vi "RS232SerialTest.vi"() -> ()   [LabVIEW 2016]
uses:
  <vilib>/FPGAPlugInAG/cRIO-9038/niLvFpga_Open_cRIO-9038.vi
  <vilib>/rvi/interface/common/dynamic/niFpgaDynamicAddResources.vi
  <vilib>/FPGAPlugInAG/Dynamic/niLvFpga_Abort_Dynamic.vi
  <vilib>/FPGAPlugInAG/Dynamic/niLvFpga_Reset_Dynamic.vi
  <vilib>/FPGAPlugInAG/Dynamic/niLvFpga_Run_Dynamic.vi
  <vilib>/Utility/error.llb/Error Cluster From Error Code.vi
  <vilib>/rvi/errors/niLvFpgaAdjustHostInterfaceError.vi
  <vilib>/FPGAPlugInAG/Dynamic/niLvFpga_Close_Dynamic.vi
  <vilib>/rvi/interface/nirviOpenFPGA/nirviOpenFPGA.xnode
  FPGA Bitfiles/Modbus_FPGATarget_RS232SerialPortT_8rmEXQNE11k.lvbitx
  RS232SerialPortTest.vi
  <vilib>/rvi/interface/nirviMethod/nirviMethod.xnode
  <vilib>/rvi/interface/nirviCloseFPGA/nirviCloseFPGA.xnode
  <vilib>/rvi/errors/niLvFpgaMergeErrorWithErrorCode.vi
  <vilib>/FPGAPlugInAG/Dynamic/niLvFpga_ReadFifo_Dynamic.vi
  <vilib>/FPGAPlugInAG/Dynamic/niLvFpga_WriteFifo_Dynamic.vi
panel:
  out "Receive":u64[](array[numeric]) format="%02x"
  in  "Send":u64[](array[numeric])=[127, 3, 0, 0, 0, 2, 206, 21] format="%02x"
  in  "Send":bool
  in  "Stop":bool
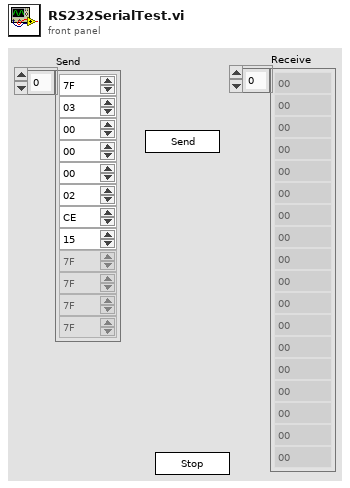
[diagram p1: front panel]
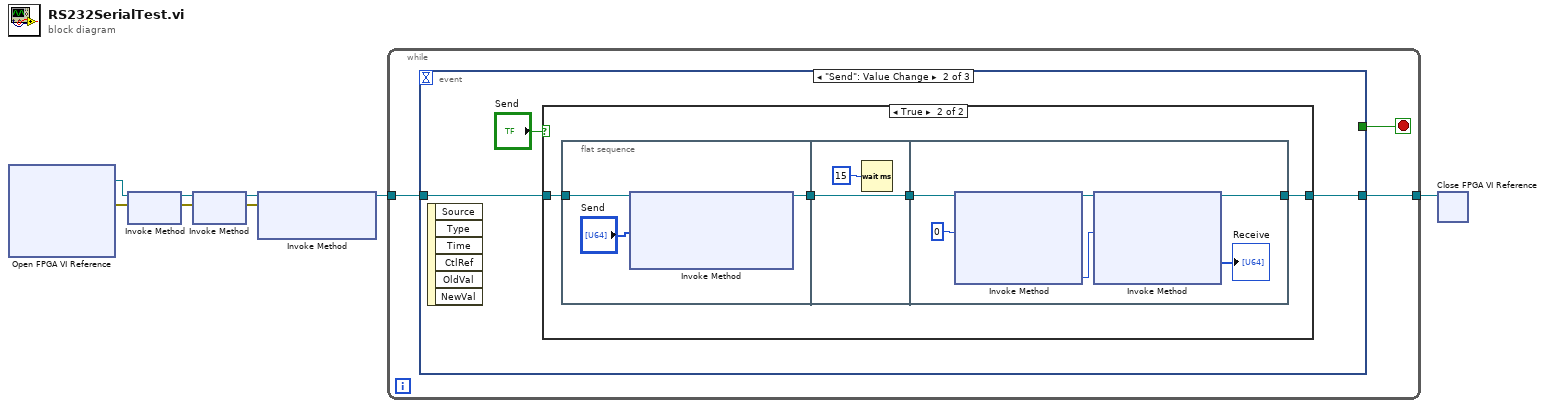
[diagram p0: block diagram]
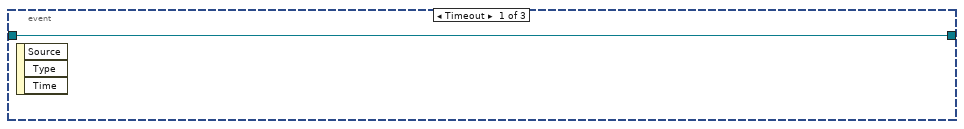
[diagram p2: hidden frame]
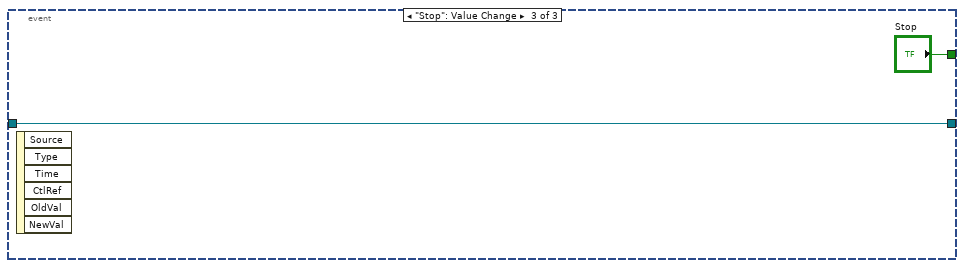
[diagram p4: hidden frame]
diagram:
  n1 = xnode "Open FPGA VI Reference"() -> ("FPGA VI Reference Out"=w8:refnum<k20>, "error out"=w5:errorcluster)  [unwired: 2 in]
  n2 = xnode "Invoke Method"("FPGA VI Reference In"=w8, "error in"=w5) -> ("FPGA VI Reference Out"=w7:refnum<k20>, "error out"=w4:errorcluster)
  n3 = xnode "Invoke Method"("FPGA VI Reference In"=w7, "error in"=w4) -> ("FPGA VI Reference Out"=w6:refnum<k20>, "error out"=w3:errorcluster)
  n4 = xnode "Invoke Method"("FPGA VI Reference In"=w6, "error in"=w3) -> ("FPGA VI Reference Out"=w2:refnum<k20>)  [unwired: 1 in, 1 out]
  n5 = while {
    tunnel: w2 -> [w11]
    tunnel: [w9] -> w1
    stop <- w10 stop-if-true
    n6 = event shown="[1] \"Send\": Value Change" {
      selector: _ -> [_ _ _]
      dyn-events: _ -> [_ _ _]
      timeout: _ -> [_ _ _]
      tunnel: w11 -> [w12 w14 w32]
      tunnel: [_ _ "Stop"] -> w10
      tunnel: [w12 w13 w32] -> w9
      event Timeout {
        n7 = event-data() -> ()  [unwired: 1 in, 3 out]
      }
      event "Send": Value Change {
        n8 = event-data() -> ()  [unwired: 1 in, 6 out]
        n9 = case shown="True" "Send" {
          tunnel: w14 -> [w16 w20]
          tunnel: [w16 w17] -> w13
          frame False {
          }
          frame True {
            n10 = flat-sequence {
              tunnel: w20 -> [w22]
              tunnel: [w21] -> w18
              tunnel: [w24] -> w19
              tunnel: w18 -> [w24]
              tunnel: w19 -> [w31]
              tunnel: [w26] -> w17
              frame #0 {
                n11 = xnode "Invoke Method"("FPGA VI Reference In"=w22, "Data"="Send") -> ("FPGA VI Reference Out"=w21:refnum<k20>)  [unwired: 2 in, 2 out]
              }
              frame #1 {
                n12 = Wait (ms)(milliseconds to wait=u32 15) -> ()  [unwired: 1 out]
              }
              frame #2 {
                n13 = xnode "Invoke Method"("FPGA VI Reference In"=w31, "Number of Elements"=u32 0) -> ("FPGA VI Reference Out"=w27:refnum<k20>, "Elements Remaining"=w29:u32)  [unwired: 2 in, 2 out]
                n14 = xnode "Invoke Method"("FPGA VI Reference In"=w27, "Number of Elements"=w29) -> ("FPGA VI Reference Out"=w26:refnum<k20>, "Data"=→"Receive":u64[])  [unwired: 2 in, 2 out]
              }
            }
          }
        }
      }
      event "Stop": Value Change {
        n15 = event-data() -> ()  [unwired: 1 in, 6 out]
      }
    }
  }
  n16 = xnode "Close FPGA VI Reference"("FPGA VI Reference In"=w1) -> ()  [unwired: 1 in, 1 out]
